vi "PID2_2V.vi"(6 "reinitialize? (F)":bool, 10 "V_afe":dbl format="%.2f", 11 "V_up":dbl format="%.2f") -> (3 "output":dbl)   [LabVIEW 2021]
uses:
  <vilib>/addons/control/pid/pid.llb/PID Advanced (DBL).vi
  <vilib>/addons/control/pid/NI_PID_pid.lvlib
panel:
  in  "PID gains":T1={"proportional gain (Kc)"=0.4, "integral time (Ti, min)"=0.05, "derivative time (Td, min)"=0.0}
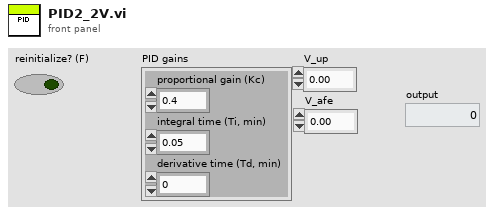
[diagram p1: front panel]
types:
  T1 = cluster{"proportional gain (Kc)":dbl, "integral time (Ti, min)":dbl, "derivative time (Td, min)":dbl}
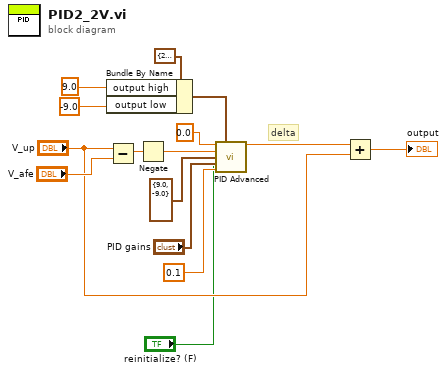
[diagram p0: block diagram]
diagram:
  # "delta"
  n1 = Bundle By Name(cluster=cluster{"output high":dbl, "output low":dbl} {"output high"=235.0, "output low"=220.0} ("output range"), "output high"=9.0 ("y"), "output low"=-9.0 ("y")) -> (w12:cluster{"output high":dbl, "output low":dbl})
  n2 = Subtract(x="V_up", y="V_afe") -> (x-y=w6:dbl)
  n3 = Negate(x=w6) -> (-x=w1:dbl)
  n4 = call-poly <vilib>:"PID Advanced.vi"("setpoint"=0.0, "output range"=w12, "process variable"=w1, "setpoint range"=cluster{"setpoint high":dbl, "setpoint low":dbl} {"setpoint high"=9.0, "setpoint low"=-9.0}, "PID gains"="PID gains", "dt (s)"=0.1, "reinitialize? (F)"="reinitialize? (F)") -> ("output"=w11:dbl)  [unwired: 7 in, 1 out]
  n5 = Add(x=w11, y="V_up") -> (x+y=→"output":dbl)
